vi "Demo.vi"() -> ()   [LabVIEW 2024]
uses:
  <vilib>/vision/NI_Vision_Development_Module.lvlib
panel:
  out "error out":errorcluster
  out "Sample":T1(plugin-control)
  in  "Path":path
  out "After":T1(plugin-control)
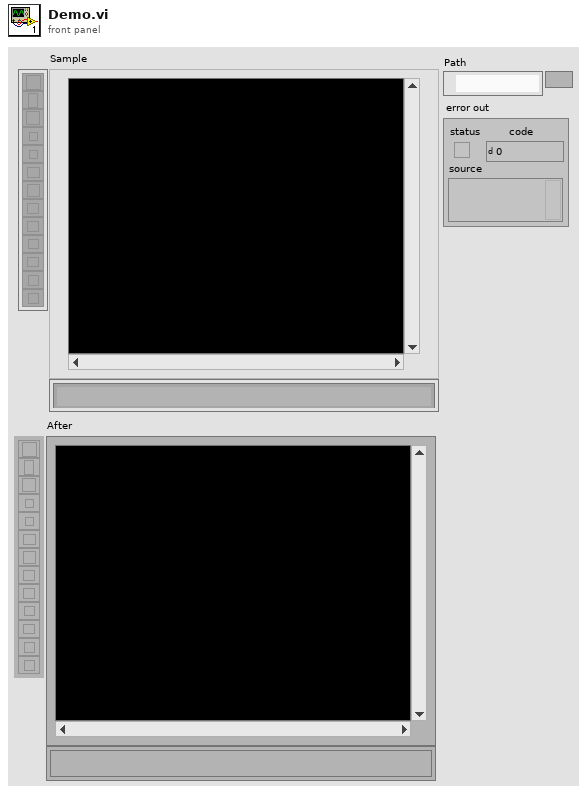
[diagram p1: front panel]
types:
  T1 = typedef "IMAQ Image.ctl" = refnum<image>
  T2 = typedef "ROI Descriptor" = cluster{"Global Rectangle":i32[], "Contours":cluster{"ID":enum32{"External", "Internal"}, "Type":u32, "Coordinates":i32[]}[]}
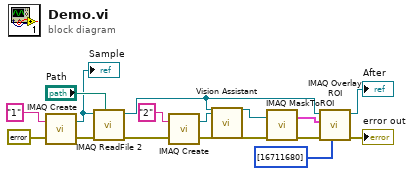
[diagram p0: block diagram]
diagram:
  n1 = call "IMAQ Create"("Image Name"="1", "error in (no error)"=errorcluster {"status"=FALSE, "code"=0, "source"=""}) -> ("New Image"=w1:T1, "error out"=w8:errorcluster)  [unwired: 3 in]
  "Sample" <- w1
  n2 = call "IMAQ ReadFile 2"("File Path"="Path", "error in (no error)"=w8, "Image"=w1) -> ("error out"=w7:errorcluster, "Image Out"=w2:T1)  [unwired: 4 in, 3 out]
  n3 = call "IMAQ Create"("Image Name"="2", "error in (no error)"=w7) -> ("New Image"=w16:T1, "error out"=w6:errorcluster)  [unwired: 3 in]
  n4 = call "Vision Assistant"("Image In"=w2, "Image Dst"=w16, "error in"=w6) -> ("Image Out"=w12:T1, "error out"=w5:errorcluster)  [unwired: 22 in, 1 out]
  n5 = call "IMAQ MaskToROI"("Image"=w12, "error in (no error)"=w5) -> ("ROI Descriptor"=w13:T2, "error out"=w4:errorcluster)  [unwired: 5 in, 1 out]
  n6 = call "IMAQ Overlay ROI"("Colors (Green)"=u32[] [16711680], "error in (no error)"=w4, "ROI Descriptor"=w13, "Image"=w2) -> ("error out"=→"error out":errorcluster, "Image Out"=→"After":T1)  [unwired: 6 in]
